vi "CanMakeSet.vi"(1 "HandCount":u16[](array[numeric])) -> (0 "CanMakeSet":bool)   [LabVIEW 2025]
panel:
  in  "VI Refnum":refnum<vi>
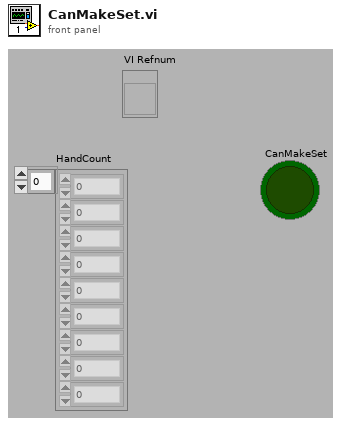
[diagram p1: front panel]
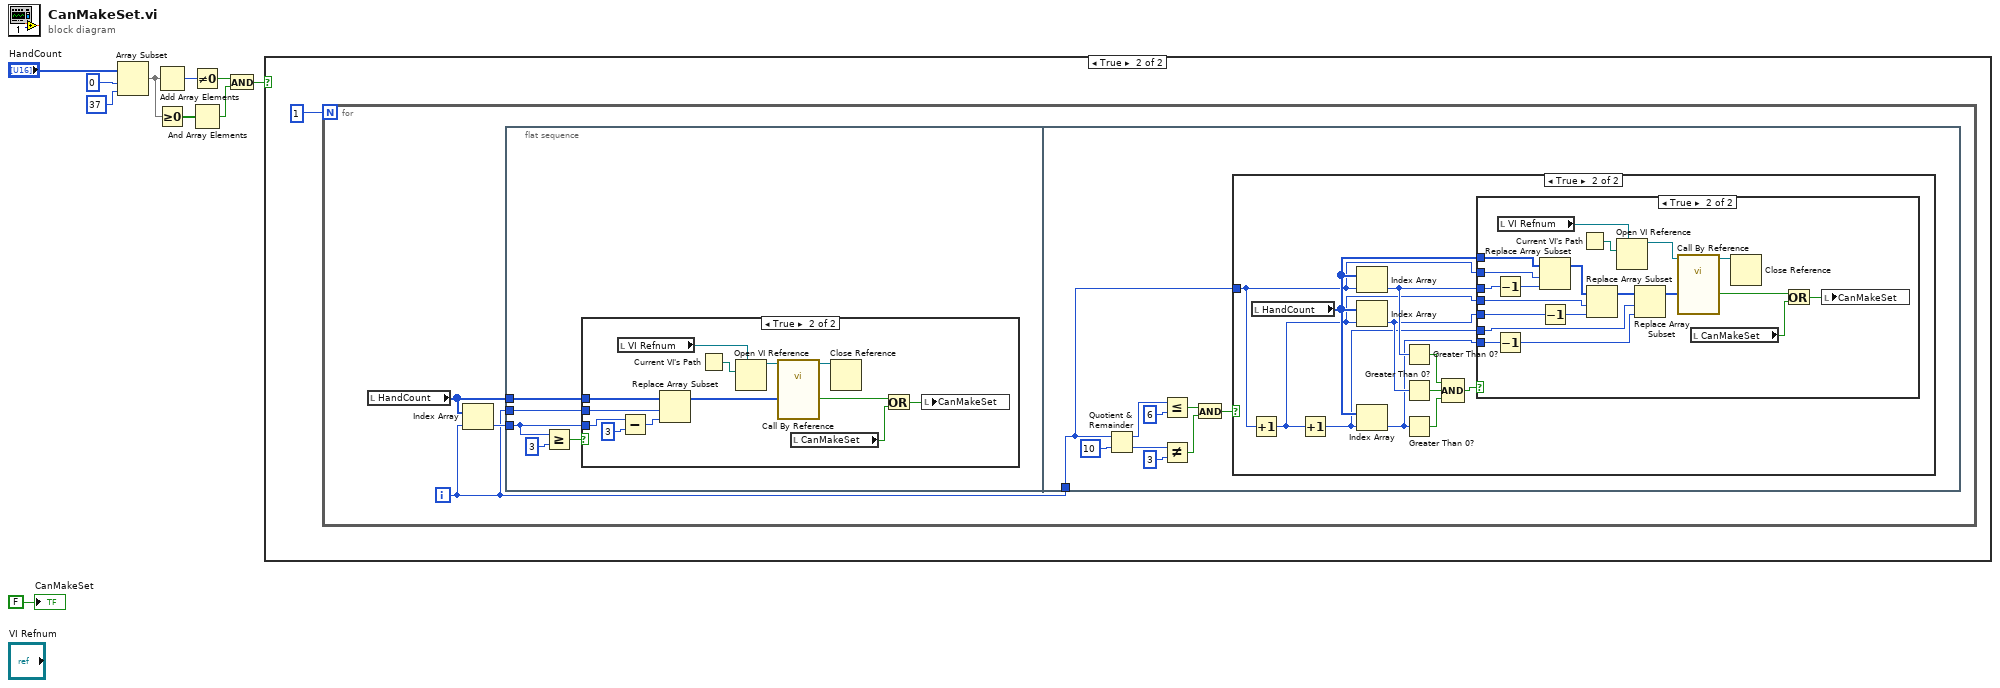
[diagram p0: block diagram]
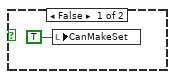
[diagram p2: hidden frame]
diagram:
  n1 = Array Subset(array="HandCount", index=0, length=37) -> (w5:u16[])
  n2 = Add Array Elements(numeric array=w5) -> (sum=w6:u16)
  n3 = Greater Or Equal To 0?(x=w5) -> (x >= 0?=w3:bool[])
  n4 = Not Equal To 0?(x=w6) -> (x != 0?=w4:bool)
  n5 = And Array Elements(Boolean array=w3) -> (logical AND=w2:bool)
  n6 = And(x=w4, y=w2) -> (x .and. y?=w1:bool)
  n7 = case shown="True" w1 {
    frame False {
      n8 = local write "CanMakeSet"(TRUE) -> ()
    }
    frame True {
      n9 = for {
        N: 1 -> [_]
        i -> [w13]
        n10 = local read "HandCount"() -> (w14:u16[])
        n11 = Index Array(array=w14, index=w13) -> (element=w15:u16)
        n12 = flat-sequence {
          tunnel: w15 -> [w16]
          tunnel: w14 -> [w18]
          tunnel: w13 -> [w17]
          tunnel: w13 -> [w35]
          frame #0 {
            n13 = Greater Or Equal?(x=w16, y=3) -> (x >= y?=w20:bool)
            n14 = case shown="True" w20 {
              tunnel: w18 -> [_ w33]
              tunnel: w17 -> [_ w32]
              tunnel: w16 -> [_ w29]
              frame False {
              }
              frame True {
                n15 = local read "VI Refnum"() -> (w21:refnum<vi>)
                n16 = Subtract(x=w29, y=3) -> (x-y=w30:i32)
                n17 = Replace Array Subset(array=w33, new element=w30, index=w32) -> (w25:u16[])
                n18 = Current VI's Path() -> (path=w28:path)
                n19 = Open VI Reference(type specifier VI Refnum (for type only)=w21, vi path=w28) -> (vi reference=w26:refnum<vi>)  [unwired: 4 in, 1 out]
                n20 = call-by-ref "?"(reference=w26, "HandCount"=w25) -> (reference out=w27:refnum<vi>, "CanMakeSet"=w24:bool)  [unwired: 1 in, 1 out]
                n21 = local read "CanMakeSet"() -> (w22:bool)
                n22 = Close Reference(reference=w27) -> ()  [unwired: 1 in, 1 out]
                n23 = Or(x=w24, y=w22) -> (x .or. y?=w23:bool)
                n24 = local write "CanMakeSet"(w23) -> ()
              }
            }
          }
          frame #1 {
            n25 = Quotient & Remainder(x=w35, y=10) -> (x-y*floor(x/y)=w41:i32, floor(x/y)=w39:i32)
            n26 = Less Or Equal?(x=w41, y=6) -> (x <= y?=w37:bool)
            n27 = Not Equal?(x=w39, y=3) -> (x != y?=w36:bool)
            n28 = And(x=w37, y=w36) -> (x .and. y?=w34:bool)
            n29 = case shown="True" w34 {
              tunnel: w35 -> [_ w45]
              frame False {
              }
              frame True {
                n30 = Increment(x=w45) -> (x+1=w49:i32)
                n31 = local read "HandCount"() -> (w52:u16[])
                n32 = Increment(x=w49) -> (x+1=w47:i32)
                n33 = Index Array(array=w52, index=w45) -> (element=w51:u16)
                n34 = Index Array(array=w52, index=w49) -> (element=w50:u16)
                n35 = Index Array(array=w52, index=w47) -> (element=w48:u16)
                n36 = Greater Than 0?(x=w51) -> (x > 0?=w53:bool)
                n37 = Greater Than 0?(x=w50) -> (x > 0?=w44:bool)
                n38 = Greater Than 0?(x=w48) -> (x > 0?=w43:bool)
                n39 = Compound Arithmetic op=AND(w53, w44, w43) -> (w46:bool)
                n40 = case shown="True" w46 {
                  tunnel: w52 -> [_ w71]
                  tunnel: w51 -> [_ w67]
                  tunnel: w50 -> [_ w66]
                  tunnel: w49 -> [_ w65]
                  tunnel: w48 -> [_ w64]
                  tunnel: w47 -> [_ w63]
                  tunnel: w45 -> [_ w54]
                  frame False {
                  }
                  frame True {
                    n41 = Decrement(x=w67) -> (x-1=w70:u16)
                    n42 = Decrement(x=w64) -> (x-1=w68:u16)
                    n43 = local read "VI Refnum"() -> (w62:refnum<vi>)
                    n44 = Replace Array Subset(array=w71, new element=w70, index=w54) -> (w73:u16[])
                    n45 = Decrement(x=w66) -> (x-1=w69:u16)
                    n46 = Current VI's Path() -> (path=w56:path)
                    n47 = Replace Array Subset(array=w73, new element=w69, index=w65) -> (w72:u16[])
                    n48 = Open VI Reference(type specifier VI Refnum (for type only)=w62, vi path=w56) -> (vi reference=w58:refnum<vi>)  [unwired: 4 in, 1 out]
                    n49 = Replace Array Subset(array=w72, new element=w68, index=w63) -> (w55:u16[])
                    n50 = call-by-ref "?"(reference=w58, "HandCount"=w55) -> (reference out=w57:refnum<vi>, "CanMakeSet"=w59:bool)  [unwired: 1 in, 1 out]
                    n51 = local read "CanMakeSet"() -> (w61:bool)
                    n52 = Close Reference(reference=w57) -> ()  [unwired: 1 in, 1 out]
                    n53 = Or(x=w59, y=w61) -> (x .or. y?=w60:bool)
                    n54 = local write "CanMakeSet"(w60) -> ()
                  }
                }
              }
            }
          }
        }
      }
    }
  }
  "CanMakeSet" <- FALSE
